vi "3 - Event Queue Decoupled from Generation.vi"() -> ()   [LabVIEW 2012]
panel:
  in  "Suspend \"B\"":bool
  in  "Suspend \"A\"":bool
  out "Messenger already dead?":errorcluster
  in  "Kill the Messenger":bool
  out "\"B\" already unregistered?":errorcluster
  out "\"A\" already unregistered?":errorcluster
  in  "Register Mailbox \"B\"":bool
  in  "Unregister Mailbox \"B\"":bool
  in  "Unregister Mailbox \"A\"":bool
  in  "Register Mailbox \"A\"":bool
  out "Messages Sent":i32
  in  "stop":bool
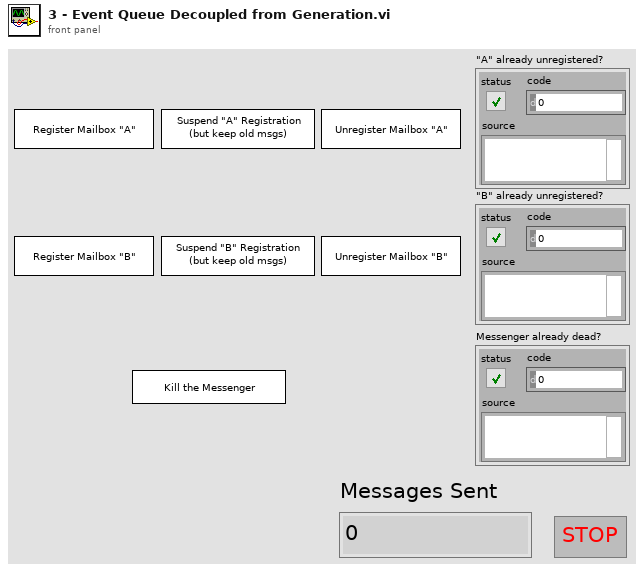
[diagram p1: front panel]
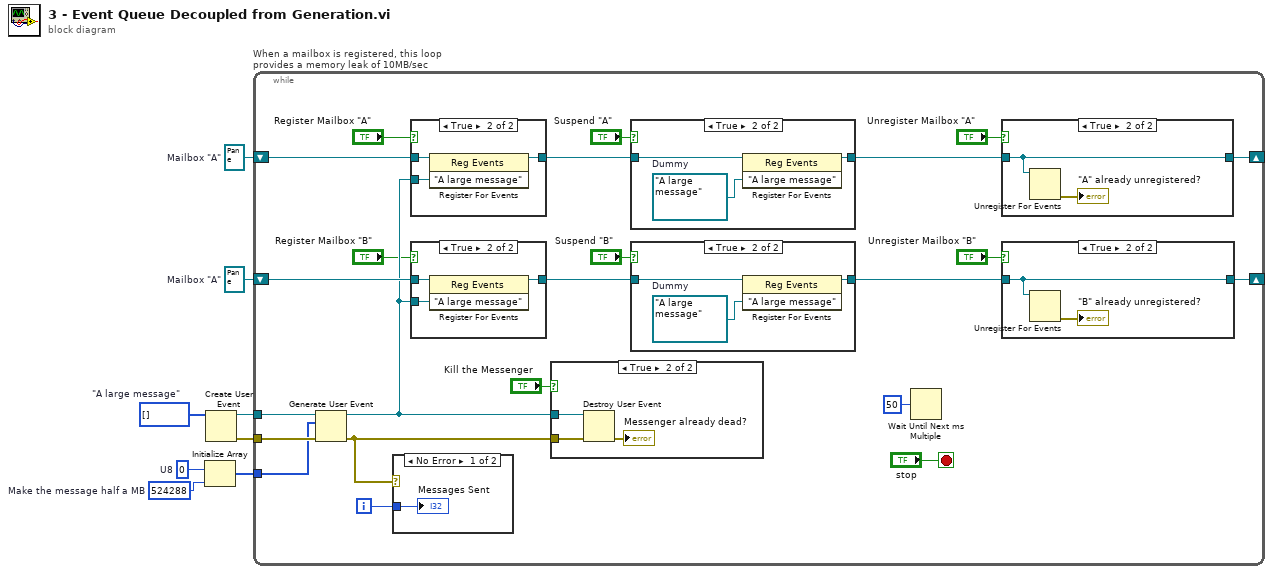
[diagram p0: block diagram]
diagram:
  w1 = refnum<event-registration> refnum  # Mailbox "A"
  w2 = refnum<event-registration> refnum  # Mailbox "A"
  w3 = u8[] []  # "A large message"
  w7 = 524288  # Make the message half a MB
  w8 = u8 0  # U8
  n1 = Initialize Array(w8, w7) -> (w4:u8[])
  n2 = Create User Event(user event datatype=w3) -> (user event=w5:refnum<user-event>, error out=w6:errorcluster)  [unwired: 1 in]
  n3 = while "When a mailbox is registered, this loop provides a memory leak of 10MB/sec" {
    tunnel: w6 -> [w30]
    tunnel: w5 -> [w31]
    tunnel: w4 -> [w28]
    shift-right: [w23] -> _
    shift-left: w2 -> [w26]
    shift-right: [w24] -> _
    shift-left: w1 -> [w25]
    i -> [w19]
    stop <- "stop" stop-if-true
    n4 = Generate User Event(user event=w31, event data cluster=w28, error in=w30) -> (user event out=w21:refnum<user-event>, error out=w20:errorcluster)
    n5 = case shown="No Error" w20 {
      tunnel: w19 -> [w40 _]
      frame No Error {
        "Messages Sent" <- w40
      }
      frame Error {
      }
    }
    n6 = case shown="True" "Register Mailbox \"A\"" {
      tunnel: w21 -> [_ w53]
      tunnel: w25 -> [w50 w52]
      tunnel: [w50 w51] -> w16
      frame False {
      }
      frame True {
        n7 = register-events(reference=w52, w53) -> (reference out=w51:refnum<event-registration>)  [unwired: 1 in, 1 out]
      }
    }
    n8 = case shown="True" "Register Mailbox \"B\"" {
      tunnel: w21 -> [_ w57]
      tunnel: w26 -> [w54 w56]
      tunnel: [w54 w55] -> w18
      frame False {
      }
      frame True {
        n9 = register-events(reference=w56, w57) -> (reference out=w55:refnum<event-registration>)  [unwired: 1 in, 1 out]
      }
    }
    n10 = case shown="True" "Kill the Messenger" {
      tunnel: w21 -> [_ w43]
      tunnel: w20 -> [_ w41]
      frame False {
      }
      frame True {
        n11 = Destroy User Event(user event=w43, error in=w41) -> (error out=→"Messenger already dead?":errorcluster)
      }
    }
    n12 = case shown="True" "Suspend \"A\"" {
      tunnel: w16 -> [w32 w35]
      tunnel: [w32 w34] -> w15
      frame False {
      }
      frame True {
        w33 = refnum<user-event> refnum  # Dummy
        n13 = register-events(reference=w35, w33) -> (reference out=w34:refnum<event-registration>)  [unwired: 1 in, 1 out]
      }
    }
    n14 = case shown="True" "Suspend \"B\"" {
      tunnel: w18 -> [w36 w39]
      tunnel: [w36 w38] -> w17
      frame False {
      }
      frame True {
        w37 = refnum<user-event> refnum  # Dummy
        n15 = register-events(reference=w39, w37) -> (reference out=w38:refnum<event-registration>)  [unwired: 1 in, 1 out]
      }
    }
    n16 = Wait Until Next ms Multiple(millisecond multiple=u32 50) -> ()  [unwired: 1 out]
    n17 = case shown="True" "Unregister Mailbox \"A\"" {
      tunnel: w15 -> [w47 w49]
      tunnel: [w47 w49] -> w24
      frame False {
      }
      frame True {
        n18 = Unregister For Events(event registration refnum=w49) -> (error out=→"\"A\" already unregistered?":errorcluster)  [unwired: 1 in]
      }
    }
    n19 = case shown="True" "Unregister Mailbox \"B\"" {
      tunnel: w17 -> [w44 w46]
      tunnel: [w44 w46] -> w23
      frame False {
      }
      frame True {
        n20 = Unregister For Events(event registration refnum=w46) -> (error out=→"\"B\" already unregistered?":errorcluster)  [unwired: 1 in]
      }
    }
  }
